vi "Read File Data.vi"(0 "VISA resource name":refnum<visa-resource-name>, 5 "File Name (\"\")":string, 7 "File Type (0 : PNG)":i32(ring) items=["PNG (Screen Image Data)", "GNL (Setting Data)", "Other File"], 9 "Save Path (\"\")":path, 11 "error in (no error)":errorcluster) -> (4 "VISA resource name out":refnum<visa-resource-name>, 15 "error out":errorcluster)   [LabVIEW 2020, in "Yokogawa GX Series.lvlib"]
doc: "Gets a file. Then saves it into the specified path.\n\nFor example:\n 1. Get *.PNG file from internal memory.\n This operation is to take a screen image data.\n Specify the File Name including the extension. e.g.: picture.PNG\n Specify the Save Path. e.g.: C:\\data\n Note: This VI cannot save screen image data when the instrument is GM10.\n 2. Get *.GNL file from internal memory.\n This operation is to get the current setting of GX series then save it to the specified file.\n Specify the File Name. e.g.: GXSetting.GDL\n Specify the Save Path. e.g.: C:\\data\n 3. Get a file from internal medium.\n This operation is to get any type of file from internal medium.\n Specify the File Name with the right position of the file in external medium and the file name. e.g.: Under the pass \"/MEM0/DATA/\" there is a file named xxx.yyy. Therefore, File Name should be set as \"/MEM0/DATA/xxx.yyy\".\n Specify the Save Path. e.g.: C:\\data\n 4. Get a file from external medium(SD card).\n This operation is to get any type of file from external medium.\n Specify the File Name with the right position(start with \"/DRV0/\"(case sensitive)) of the file in external medium and the file name. e.g.: Under the pass \"/DRV0/\" there is a file named xxx.yyy. Therefore, File Name should be set as \"/DRV0/xxx.yyy\".\n Specify the Save Path. e.g.: C:\\data"
uses:
  <instrlib>/Yokogawa GX Series/Yokogawa GX Series.lvlib
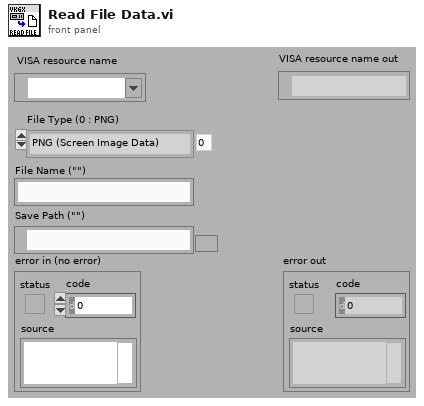
[diagram p1: front panel]
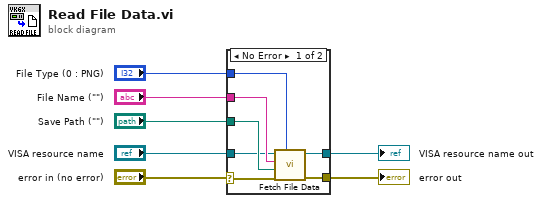
[diagram p0: block diagram]
diagram:
  n1 = case shown="No Error" "error in (no error)" {
    selector: "error in (no error)" -> [w8 w15]
    tunnel: "Save Path (\"\")" -> [w14 _]
    tunnel: [w13 w16] -> w6
    tunnel: [w12 w15] -> w5
    tunnel: "File Name (\"\")" -> [w11 _]
    tunnel: "VISA resource name" -> [w10 w16]
    tunnel: "File Type (0 : PNG)" -> [w9 _]
    frame No Error {
      n2 = call <instrlib>:"Fetch File Data.vi"("File Type (0 : PNG)"=w9, "error in (no error)"=w8, "Save Path (\"\")"=w14, "File Name (\"\")"=w11, "VISA resource name"=w10) -> ("error out"=w12:errorcluster, "VISA resource name out"=w13:refnum<visa-resource-name>)  [unwired: 5 in]
    }
    frame Error {
    }
  }
  "error out" <- w5
  "VISA resource name out" <- w6
